vi "Serial Port Read.vi"(2 "requested byte count":u32, 3 "port number":i32) -> (0 "error code":i32 format="%x", 1 "string read":string)   [LabVIEW 2013]
doc: "Reads the number of characters specified by <B>requested byte count</B> from the serial port indicated in <B>port number</B>."
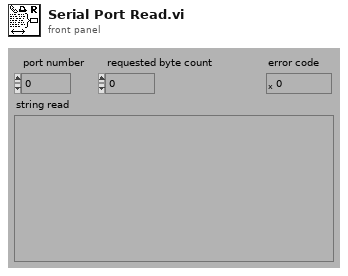
[diagram p1: front panel]
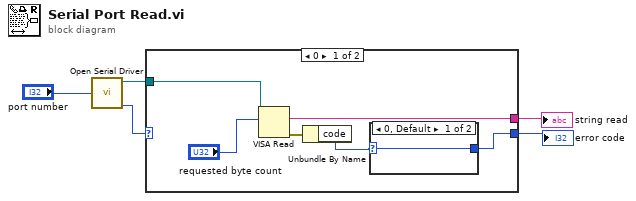
[diagram p0: block diagram]
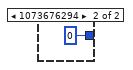
[diagram p2: hidden frame]
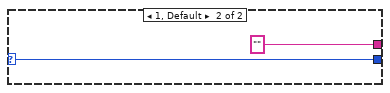
[diagram p3: hidden frame]
diagram:
  n1 = call "Open Serial Driver.vi"("port number"="port number") -> ("input refnum"=w3:refnum<visa-resource-name>, "output error"=w4:i32)  [unwired: 2 out]
  n2 = case shown="0" w4 {
    selector: w4 -> [_ w15]
    tunnel: w3 -> [w11 _]
    tunnel: [w9 "" ("read buffer")] -> w2
    tunnel: [w6 w15] -> w1
    frame 0 {
      n3 = VISA Read(VISA resource name=w11, byte count="requested byte count") -> (read buffer=w9:string, error out=w8:errorcluster)  [unwired: 1 in, 2 out]
      n4 = Unbundle By Name(w8) -> ("code"=w7:i32)
      n5 = case shown="0, Default" w7 {
        selector: w7 -> [w12 _]
        tunnel: [w12 0 ("code")] -> w6
        frame 0, Default {
        }
        frame 1073676294 {
        }
      }
    }
    frame 1, Default {
    }
  }
  "string read" <- w2
  "error code" <- w1
